vi "Plug in names.vi"() -> (0 "Array":string[](array[string]))   [LabVIEW 2022 SP3]
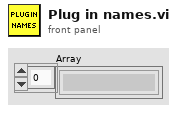
[diagram p1: front panel]
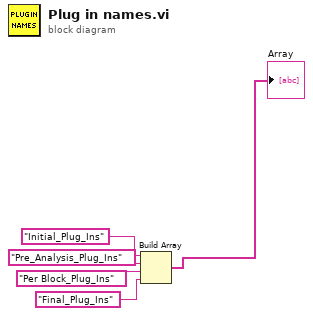
[diagram p0: block diagram]
diagram:
  n1 = Build Array("Initial_Plug_Ins", "Pre_Analysis_Plug_Ins", "Per Block_Plug_Ins", "Final_Plug_Ins") -> (→"Array":string[])
